vi "CalculateBMonly.vi"() -> ()   [LabVIEW 2016]
uses:
  <vilib>/Analysis/baseanly.llb/Mean (DBL).vi
  <vilib>/Utility/file.llb/Read Delimited Spreadsheet (string).vi
  <vilib>/Utility/file.llb/Write Delimited Spreadsheet (DBL).vi
  <vilib>/Analysis/NI_AALBase.lvlib
panel:
  in  "Save XY plot":bool
  out "XYplot":path
  in  "complete":bool
  in  "recalculate":bool
  in  "Save BM":bool
  out "good aoi":i32[](array[numeric])
  out "yBM":dbl[](array[numeric])
  out "xBM":dbl[](array[numeric])
  in  "Tab Control":enum32{"Files data", "Each file data"}(tab)
  out "N=":i32
  out "Filenames":string[](array[string])
  out "# of Frames":dbl[](array[numeric])
  out "# of AOI":dbl[](array[numeric])
  out "useful AOIs":dbl[](array[numeric])
  out "% of useful AOIs":dbl
  out "tt # of useful AOIs":i32
  out "tt # of AOIs":i32
  out "?":T1(graph)
  out "Xm=":dbl format="%0.2f"
  out "Ym=":dbl format="%0.2f"
  in  "Intervals":i32=10
  out "?":T1(graph)
  out "useful Aois (each file)":i32
  out "XY plot":T2
  in  "mode":enum32{"slide by slide", "delay"}(tab)=enum."delay"
  in  "next":bool
  in  "Run over":bool
  in  "second":dbl
  in  "run over":bool
  out "File":string
  in  "nm/pixel":dbl=72.5
  in  "±":dbl=50.0
  in  "BM":dbl=50.0
  out "BM lower limit":dbl
  out "BM upper limit":dbl
  in  "R should less than":dbl=0.2
  in  "lower limit":dbl=0.85
  in  "upper limit":dbl=1.15
  in  "BM range":bool=TRUE
  in  "Relation coefficient":bool
  in  "rotate?":bool
  in  "x/y":bool=TRUE
  out "all y position\n(pixel)":dbl[][](array[numeric])
  out "all x position\n(pixel)":dbl[][](array[numeric])
  out "# of frames":dbl
  out "# of AOIs":dbl
  out "Tandem Yi position":dbl[](array[numeric])
  out "Tandem Xi position":dbl[](array[numeric])
  out "path out":path
  in  "Path Folder":path
  out "XY Graph 2":cluster{dbl[], dbl[]}(graph)
  # "nm"
  # "nm"
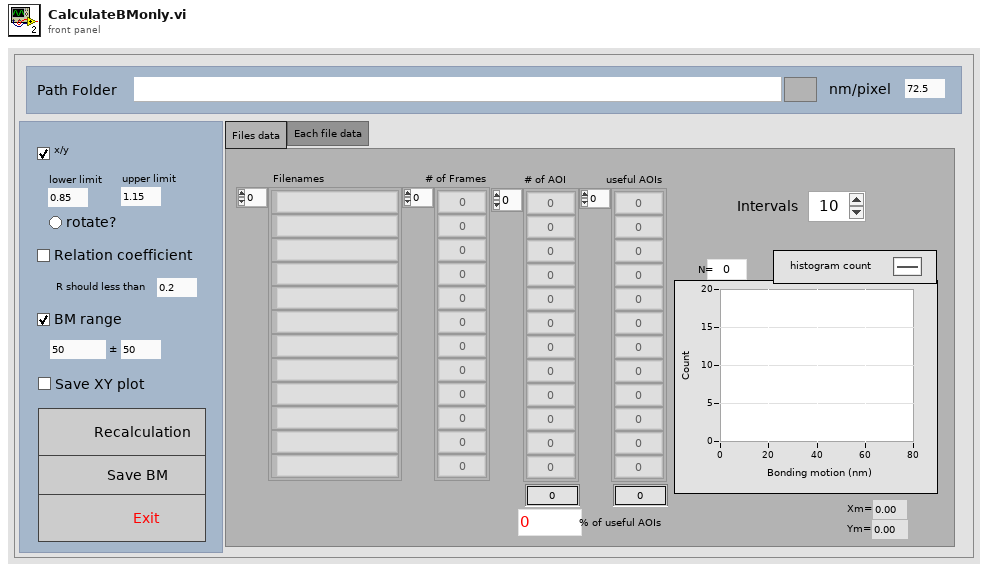
[diagram p1: front panel]
types:
  T1 = cluster{"X Values":dbl[], "Histogram: h(x)":i32[]}
  T2 = cluster{" X-Y plot":cluster{dbl[], dbl[]}, "Aoi":i32, "X BM":dbl, "Y BM":dbl}
  T3 = cluster{cluster{dbl[], dbl[]}, i32, "x standard deviation":dbl, "y standard deviation":dbl}
  T4 = typedef "imagedata.ctl" = cluster{"image type":i32, "image depth":i32, "image":u8[], "mask":u8[], "colors":u32[], "Rectangle":cluster{"left":i16, "top":i16, "right":i16, "bottom":i16}}
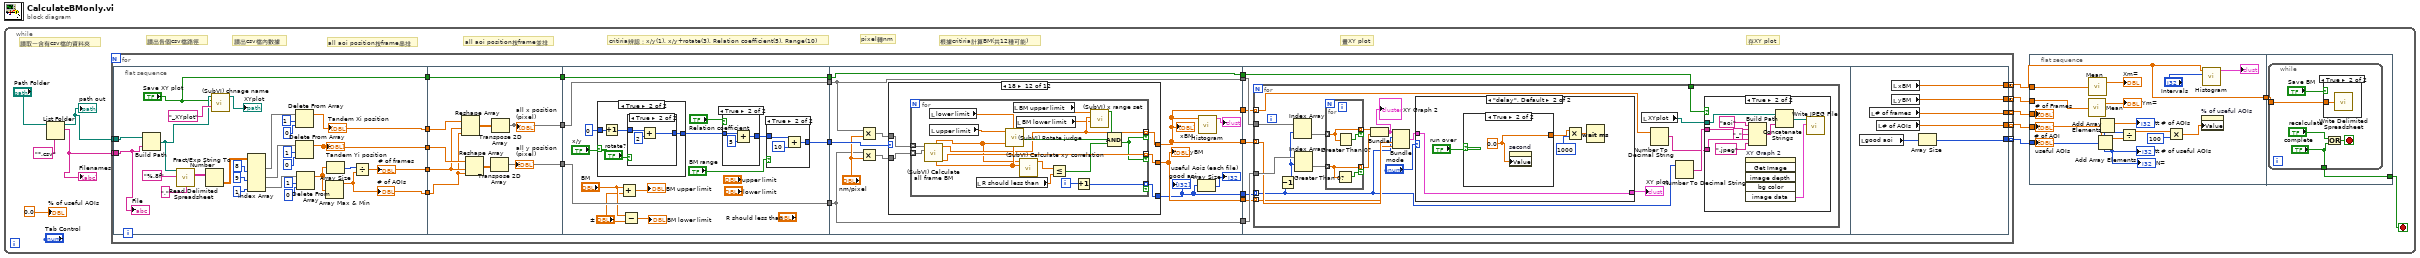
[diagram p0: block diagram]
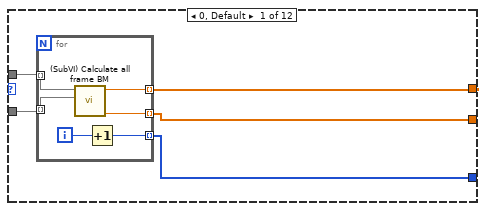
[diagram p7: hidden frame]
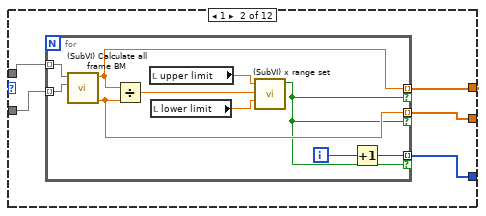
[diagram p8: hidden frame]
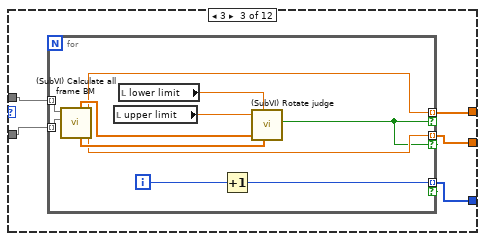
[diagram p9: hidden frame]
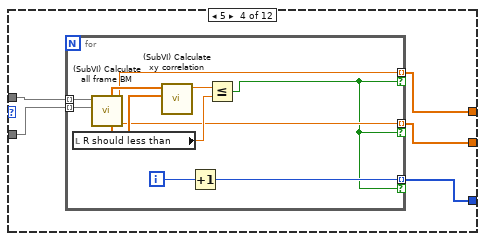
[diagram p10: hidden frame]
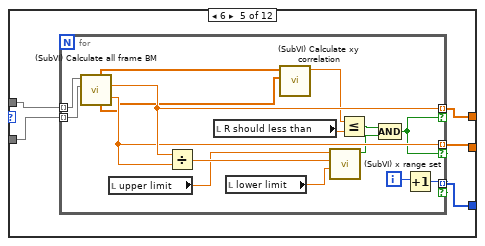
[diagram p11: hidden frame]
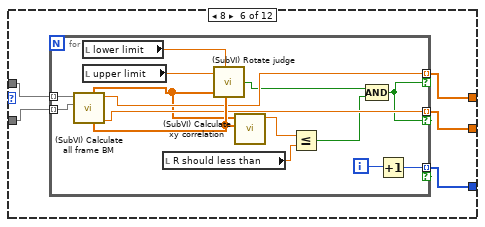
[diagram p12: hidden frame]
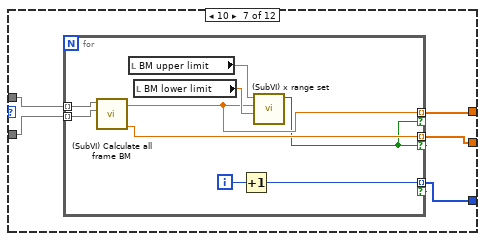
[diagram p13: hidden frame]
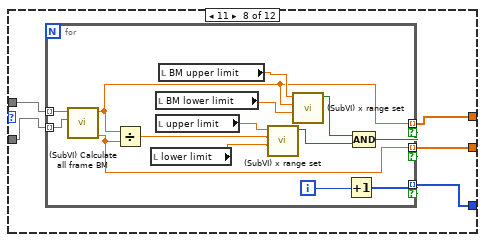
[diagram p14: hidden frame]
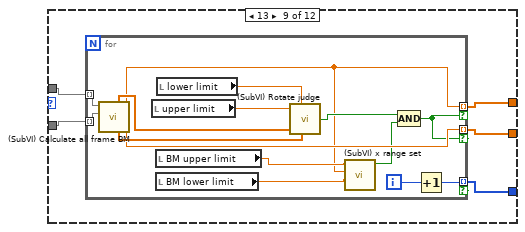
[diagram p15: hidden frame]
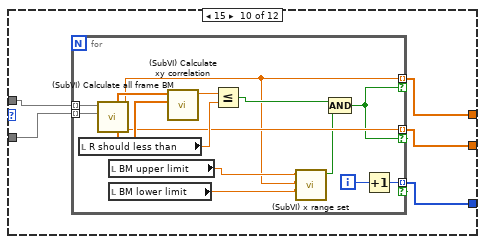
[diagram p16: hidden frame]
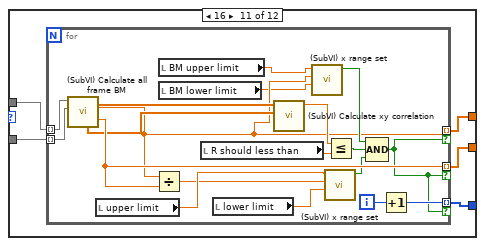
[diagram p17: hidden frame]
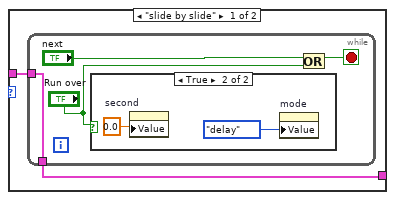
[diagram p19: hidden frame]
diagram:
  n1 = while {
    stop <- w2 stop-if-true
    # "存XY plot"
    # "畫XY plot"
    # "pixel轉nm"
    # "根據critiria計算BM(共12種可能)"
    # "critiria辨認：x/y(1), x/y+rotate(3), Relation coefficient(5), Range(10)"
    # "all aoi position按frame並排"
    # "all aoi position按frame串排"
    # "讀出csv檔內數據"
    # "讀出各個csv檔路徑"
    # "讀取一含有csv檔的資料夾"
    n2 = List Folder(path="Path Folder", pattern="*.csv") -> (path out=w9:path, filenames=w3:string[])  [unwired: 2 in, 2 out]
    "path out" <- w9
    "Filenames" <- w3
    n3 = for {
      tunnel: w9 -> [w51]
      tunnel: w3 -> [w50] mode=indexing
      tunnel: [w49] -> w4 mode=concatenating
      tunnel: [w48] -> w7 mode=concatenating
      tunnel: [w44] -> w5 mode=indexing
      tunnel: [w43] -> w8 mode=indexing
      tunnel: [w42] -> w6 mode=indexing
      n4 = flat-sequence {
        tunnel: [w88] -> w60
        tunnel: [w87] -> w59
        tunnel: [w86] -> w58
        tunnel: [w85] -> w57
        tunnel: w51 -> [w84]
        tunnel: w50 -> [w65]
        tunnel: ["Save XY plot"] -> w37
        tunnel: w60 -> [w97]
        tunnel: w59 -> [w96]
        tunnel: w58 -> [w95]
        tunnel: w57 -> [w94]
        tunnel: [w93] -> w56
        tunnel: [w92] -> w55
        tunnel: [w89] -> w38
        tunnel: w37 -> [w89]
        tunnel: w56 -> [w104]
        tunnel: w55 -> [w103]
        tunnel: [w105] -> w54
        tunnel: [w104] -> w53
        tunnel: [w103] -> w52
        tunnel: [w98] -> w39
        tunnel: w38 -> [w98]
        tunnel: w54 -> [w140]
        tunnel: w53 -> [w136]
        tunnel: w52 -> [w135]
        tunnel: [w130] -> w47
        tunnel: [w136] -> w46
        tunnel: [w135] -> w45
        tunnel: [w132] -> w41
        tunnel: [w134] -> w40
        tunnel: w39 -> [w133]
        tunnel: [w133] -> w36
        tunnel: [w132] -> w35
        tunnel: w40 -> [w362]
        tunnel: w41 -> [w363]
        tunnel: w45 -> [w365]
        tunnel: w46 -> [w366]
        tunnel: w47 -> [w364]
        tunnel: w36 -> [w361]
        tunnel: w35 -> [w360]
        tunnel: [w418] -> w48
        tunnel: [w419] -> w49
        tunnel: [w415] -> w44
        tunnel: [w417] -> w43
        tunnel: [w416] -> w42
        frame #0 {
          n5 = Build Path(base path=w84, name or relative path=w65) -> (appended path=w62:path)
          n6 = call-poly <vilib>:"Read Delimited Spreadsheet.vi"("file path (dialog if empty)"=w62, "format (%s)"="%.8f", "delimiter (\\t)"="," ("delimiter (\\t)")) -> ("all rows"=w81:string[][])  [unwired: 7 in, 5 out]
          n7 = Fract/Exp String To Number(string=w81) -> (number=w80:dbl[][])  [unwired: 3 in, 1 out]
          n8 = call "(SubVI) chnage name.vi"("replace \".csv\" to"="_XYplot" ("replace string (\"\")"), "Create path?"="Save XY plot", "Folder path"=w62) -> ("created path"=→"XYplot":path)  [unwired: 8 in]
          n9 = Index Array(array=w80, index (col) #1=8 ("disabled index (col)"), index (col) #2=9 ("index (col)"), index (col) #3=1 ("index (col)")) -> (element #1=w70:dbl[], element #2=w69:dbl[], element #3=w68:dbl[])  [unwired: 3 in]
          n10 = Delete From Array(array=w70, length=1, index=0) -> (array with subset deleted=w88:dbl[])  [unwired: 1 out]
          "Tandem Xi position" <- w88
          n11 = Delete From Array(array=w69, length=1, index=0) -> (array with subset deleted=w87:dbl[])  [unwired: 1 out]
          "Tandem Yi position" <- w87
          n12 = Delete From Array(array=w68, length=1, index=0) -> (array with subset deleted=w67:dbl[])  [unwired: 1 out]
          n13 = Array Max & Min(array=w67) -> (max value=w85:dbl)  [unwired: 3 out]
          "# of AOIs" <- w85
          n14 = Array Size(array=w67) -> (size(s)=w66:i32)
          n15 = Divide(x=w66, y=w85) -> (x/y=w86:dbl)
          "# of frames" <- w86
          "File" <- w65
        }
        frame #1 {
          n16 = Reshape Array(w97, w95, w94) -> (w91:dbl[][])
          n17 = Reshape Array(w96, w95, w94) -> (w90:dbl[][])
          n18 = Transpose 2D Array(2D array=w90) -> (transposed array=w92:dbl[][])
          "all y position\n(pixel)" <- w92
          n19 = Transpose 2D Array(2D array=w91) -> (transposed array=w93:dbl[][])
          "all x position\n(pixel)" <- w93
        }
        frame #2 {
          n20 = case shown="True" "x/y" {
            tunnel: 0 -> [w120 w124]
            tunnel: [w120 w121] -> w108
            frame False {
            }
            frame True {
              n21 = Increment(x=w124) -> (x+1=w122:i32)
              n22 = case shown="True" "rotate?" {
                tunnel: w122 -> [w125 w127]
                tunnel: [w125 w126] -> w121
                frame False {
                }
                frame True {
                  n23 = Add(x=w127, y=2) -> (x+y=w126:i32)
                }
              }
            }
          }
          n24 = Add(x="BM", y="±") -> (x+y=→"BM upper limit":dbl)
          n25 = Subtract(x="BM", y="±") -> (x-y=→"BM lower limit":dbl)
          n26 = case shown="True" "Relation coefficient" {
            tunnel: w108 -> [w116 w118]
            tunnel: [w116 w117] -> w111
            frame False {
            }
            frame True {
              n27 = Add(x=w118, y=5) -> (x+y=w117:i32)
            }
          }
          n28 = case shown="True" "BM range" {
            tunnel: w111 -> [w112 w114]
            tunnel: [w112 w113] -> w105
            frame False {
            }
            frame True {
              n29 = Add(x=w114, y=10) -> (x+y=w113:i32)
            }
          }
        }
        frame #3 {
          n30 = Multiply(x=w136, y="nm/pixel") -> (x*y=w138:dbl[][])
          n31 = Multiply(x=w135, y="nm/pixel") -> (x*y=w137:dbl[][])
          n32 = case shown="18" w140 {
            tunnel: w138 -> [w145 w156 w171 w187 w203 w224 w244 w258 w277 w297 w317 w341]
            tunnel: w137 -> [w144 w155 w170 w186 w202 w223 w243 w257 w276 w296 w316 w340]
            tunnel: [w143 w154 w169 w185 w201 w222 w242 w256 w275 w295 w315 w339] -> w132
            tunnel: [w142 w153 w168 w184 w200 w221 w241 w255 w274 w294 w314 w338] -> w134
            tunnel: [w141 w152 w167 w183 w199 w220 w240 w254 w273 w293 w313 w337] -> w130
            frame 0, Default {
              n33 = for {
                tunnel: w145 -> [w151] mode=indexing
                tunnel: w144 -> [w150] mode=indexing
                tunnel: [w149] -> w143 mode=indexing
                tunnel: [w148] -> w142 mode=indexing
                tunnel: [w146] -> w141 mode=indexing
                i -> [w147]
                n34 = call "(SubVI) Calculate all frame BM.vi"("y position (pixel)"=w150, "x position (pixel)"=w151) -> ("y standard deviation"=w148:dbl, "x standard deviation"=w149:dbl)  [unwired: 6 in, 2 out]
                n35 = Increment(x=w147) -> (x+1=w146:i32)
              }
            }
            frame 1 {
              n36 = for {
                tunnel: [w166] -> w154 mode=indexing if=w158
                tunnel: [w165] -> w153 mode=indexing if=w158
                tunnel: w156 -> [w164] mode=indexing
                tunnel: w155 -> [w163] mode=indexing
                tunnel: [w157] -> w152 mode=indexing if=w158
                i -> [w159]
                n37 = call "(SubVI) Calculate all frame BM.vi"("y position (pixel)"=w163, "x position (pixel)"=w164) -> ("y standard deviation"=w165:dbl, "x standard deviation"=w166:dbl)  [unwired: 6 in, 2 out]
                n38 = Divide(x=w166, y=w165) -> (x/y=w161:dbl)
                n39 = local read "upper limit"() -> (w162:dbl)
                n40 = local read "lower limit"() -> (w160:dbl)
                n41 = call "(SubVI) x range set.vi"("lower limit"=w160, "x"=w161, "upper limit"=w162) -> ("Boolean"=w158:bool)  [unwired: 8 in]
                n42 = Increment(x=w159) -> (x+1=w157:i32)
              }
            }
            frame 3 {
              n43 = for {
                tunnel: w171 -> [w182] mode=indexing
                tunnel: w170 -> [w181] mode=indexing
                tunnel: [w176] -> w169 mode=indexing if=w172
                tunnel: [w175] -> w168 mode=indexing if=w172
                tunnel: [w173] -> w167 mode=indexing if=w172
                i -> [w174]
                n44 = call "(SubVI) Calculate all frame BM.vi"("y position (pixel)"=w181, "x position (pixel)"=w182) -> ("y standard deviation"=w175:dbl, "x standard deviation"=w176:dbl, "y position (delete y fit error)"=w179:dbl[], "x position (delete x fit error)"=w180:dbl[])  [unwired: 6 in]
                n45 = local read "upper limit"() -> (w178:dbl)
                n46 = local read "lower limit"() -> (w177:dbl)
                n47 = Increment(x=w174) -> (x+1=w173:i32)
                n48 = call "(SubVI) Rotate judge.vi"("x/y upper limit"=w178, "x/y lower limit"=w177, "x position (delete y fit error)"=w180, "y position (delete y fit error)"=w179) -> ("x = y?"=w172:bool)  [unwired: 1 in]
              }
            }
            frame 5 {
              n49 = for {
                tunnel: w187 -> [w198] mode=indexing
                tunnel: w186 -> [w197] mode=indexing
                tunnel: [w192] -> w185 mode=indexing if=w188
                tunnel: [w191] -> w184 mode=indexing if=w188
                tunnel: [w189] -> w183 mode=indexing if=w188
                i -> [w190]
                n50 = local read "R should less than"() -> (w193:dbl)
                n51 = call "(SubVI) Calculate all frame BM.vi"("y position (pixel)"=w197, "x position (pixel)"=w198) -> ("y standard deviation"=w191:dbl, "x standard deviation"=w192:dbl, "y position (delete y fit error)"=w195:dbl[], "x position (delete x fit error)"=w196:dbl[])  [unwired: 6 in]
                n52 = call "(SubVI) Calculate xy correlation.vi"("y position (delete y fit error)"=w195, "x position (delete x fit error)"=w196) -> ("Numeric"=w194:dbl)  [unwired: 9 in]
                n53 = Increment(x=w190) -> (x+1=w189:i32)
                n54 = Less Or Equal?(x=w194, y=w193) -> (x <= y?=w188:bool)
              }
            }
            frame 6 {
              n55 = for {
                tunnel: w203 -> [w219] mode=indexing
                tunnel: w202 -> [w218] mode=indexing
                tunnel: [w217] -> w201 mode=indexing if=w204
                tunnel: [w216] -> w200 mode=indexing if=w204
                tunnel: [w205] -> w199 mode=indexing if=w204
                i -> [w206]
                n56 = call "(SubVI) Calculate all frame BM.vi"("y position (pixel)"=w218, "x position (pixel)"=w219) -> ("y standard deviation"=w216:dbl, "x standard deviation"=w217:dbl, "y position (delete y fit error)"=w212:dbl[], "x position (delete x fit error)"=w213:dbl[])  [unwired: 6 in]
                n57 = local read "upper limit"() -> (w208:dbl)
                n58 = Divide(x=w217, y=w216) -> (x/y=w209:dbl)
                n59 = local read "R should less than"() -> (w214:dbl)
                n60 = local read "lower limit"() -> (w207:dbl)
                n61 = call "(SubVI) Calculate xy correlation.vi"("y position (delete y fit error)"=w212, "x position (delete x fit error)"=w213) -> ("Numeric"=w215:dbl)  [unwired: 9 in]
                n62 = call "(SubVI) x range set.vi"("lower limit"=w207, "x"=w209, "upper limit"=w208) -> ("Boolean"=w211:bool)  [unwired: 8 in]
                n63 = Less Or Equal?(x=w215, y=w214) -> (x <= y?=w210:bool)
                n64 = Compound Arithmetic op=AND(w210, w211) -> (w204:bool)
                n65 = Increment(x=w206) -> (x+1=w205:i32)
              }
            }
            frame 8 {
              n66 = for {
                tunnel: w224 -> [w239] mode=indexing
                tunnel: w223 -> [w238] mode=indexing
                tunnel: [w232] -> w222 mode=indexing if=w226
                tunnel: [w231] -> w221 mode=indexing if=w226
                tunnel: [w227] -> w220 mode=indexing if=w226
                i -> [w228]
                n67 = call "(SubVI) Calculate all frame BM.vi"("y position (pixel)"=w238, "x position (pixel)"=w239) -> ("y standard deviation"=w231:dbl, "x standard deviation"=w232:dbl, "y position (delete y fit error)"=w237:dbl[], "x position (delete x fit error)"=w225:dbl[])  [unwired: 6 in]
                n68 = local read "lower limit"() -> (w235:dbl)
                n69 = local read "upper limit"() -> (w236:dbl)
                n70 = local read "R should less than"() -> (w233:dbl)
                n71 = call "(SubVI) Rotate judge.vi"("x/y upper limit"=w236, "x/y lower limit"=w235, "x position (delete y fit error)"=w225, "y position (delete y fit error)"=w237) -> ("x = y?"=w230:bool)  [unwired: 1 in]
                n72 = call "(SubVI) Calculate xy correlation.vi"("y position (delete y fit error)"=w237, "x position (delete x fit error)"=w225) -> ("Numeric"=w234:dbl)  [unwired: 9 in]
                n73 = Less Or Equal?(x=w234, y=w233) -> (x <= y?=w229:bool)
                n74 = Compound Arithmetic op=AND(w230, w229) -> (w226:bool)
                n75 = Increment(x=w228) -> (x+1=w227:i32)
              }
            }
            frame 10 {
              n76 = for {
                tunnel: w244 -> [w253] mode=indexing
                tunnel: w243 -> [w252] mode=indexing
                tunnel: [w248] -> w242 mode=indexing if=w245
                tunnel: [w251] -> w241 mode=indexing if=w245
                tunnel: [w246] -> w240 mode=indexing if=w245
                i -> [w247]
                n77 = call "(SubVI) Calculate all frame BM.vi"("y position (pixel)"=w252, "x position (pixel)"=w253) -> ("y standard deviation"=w251:dbl, "x standard deviation"=w248:dbl)  [unwired: 6 in, 2 out]
                n78 = local read "BM upper limit"() -> (w250:dbl)
                n79 = local read "BM lower limit"() -> (w249:dbl)
                n80 = Increment(x=w247) -> (x+1=w246:i32)
                n81 = call "(SubVI) x range set.vi"("lower limit"=w249, "x"=w248, "upper limit"=w250) -> ("Boolean"=w245:bool)  [unwired: 8 in]
              }
            }
            frame 11 {
              n82 = for {
                tunnel: w258 -> [w272] mode=indexing
                tunnel: w257 -> [w271] mode=indexing
                tunnel: [w267] -> w256 mode=indexing if=w259
                tunnel: [w270] -> w255 mode=indexing if=w259
                tunnel: [w260] -> w254 mode=indexing if=w259
                i -> [w261]
                n83 = call "(SubVI) Calculate all frame BM.vi"("y position (pixel)"=w271, "x position (pixel)"=w272) -> ("y standard deviation"=w270:dbl, "x standard deviation"=w267:dbl)  [unwired: 6 in, 2 out]
                n84 = Divide(x=w267, y=w270) -> (x/y=w263:dbl)
                n85 = local read "lower limit"() -> (w262:dbl)
                n86 = local read "BM lower limit"() -> (w266:dbl)
                n87 = local read "upper limit"() -> (w265:dbl)
                n88 = local read "BM upper limit"() -> (w268:dbl)
                n89 = call "(SubVI) x range set.vi"("lower limit"=w262, "x"=w263, "upper limit"=w265) -> ("Boolean"=w264:bool)  [unwired: 8 in]
                n90 = call "(SubVI) x range set.vi"("lower limit"=w266, "x"=w267, "upper limit"=w268) -> ("Boolean"=w269:bool)  [unwired: 8 in]
                n91 = Increment(x=w261) -> (x+1=w260:i32)
                n92 = Compound Arithmetic op=AND(w269, w264) -> (w259:bool)
              }
            }
            frame 13 {
              n93 = for {
                tunnel: w277 -> [w292] mode=indexing
                tunnel: w276 -> [w291] mode=indexing
                tunnel: [w282] -> w275 mode=indexing if=w278
                tunnel: [w286] -> w274 mode=indexing if=w278
                tunnel: [w279] -> w273 mode=indexing if=w278
                i -> [w280]
                n94 = call "(SubVI) Calculate all frame BM.vi"("y position (pixel)"=w291, "x position (pixel)"=w292) -> ("y standard deviation"=w286:dbl, "x standard deviation"=w282:dbl, "y position (delete y fit error)"=w289:dbl[], "x position (delete x fit error)"=w290:dbl[])  [unwired: 6 in]
                n95 = local read "upper limit"() -> (w288:dbl)
                n96 = local read "BM upper limit"() -> (w283:dbl)
                n97 = local read "BM lower limit"() -> (w281:dbl)
                n98 = local read "lower limit"() -> (w287:dbl)
                n99 = call "(SubVI) Rotate judge.vi"("x/y upper limit"=w288, "x/y lower limit"=w287, "x position (delete y fit error)"=w290, "y position (delete y fit error)"=w289) -> ("x = y?"=w285:bool)  [unwired: 1 in]
                n100 = call "(SubVI) x range set.vi"("lower limit"=w281, "x"=w282, "upper limit"=w283) -> ("Boolean"=w284:bool)  [unwired: 8 in]
                n101 = Compound Arithmetic op=AND(w285, w284) -> (w278:bool)
                n102 = Increment(x=w280) -> (x+1=w279:i32)
              }
            }
            frame 15 {
              n103 = for {
                tunnel: w297 -> [w312] mode=indexing
                tunnel: w296 -> [w311] mode=indexing
                tunnel: [w302] -> w295 mode=indexing if=w298
                tunnel: [w306] -> w294 mode=indexing if=w298
                tunnel: [w299] -> w293 mode=indexing if=w298
                i -> [w300]
                n104 = local read "R should less than"() -> (w307:dbl)
                n105 = call "(SubVI) Calculate all frame BM.vi"("y position (pixel)"=w311, "x position (pixel)"=w312) -> ("y standard deviation"=w306:dbl, "x standard deviation"=w302:dbl, "y position (delete y fit error)"=w309:dbl[], "x position (delete x fit error)"=w310:dbl[])  [unwired: 6 in]
                n106 = local read "BM upper limit"() -> (w303:dbl)
                n107 = local read "BM lower limit"() -> (w301:dbl)
                n108 = call "(SubVI) Calculate xy correlation.vi"("y position (delete y fit error)"=w309, "x position (delete x fit error)"=w310) -> ("Numeric"=w308:dbl)  [unwired: 9 in]
                n109 = Less Or Equal?(x=w308, y=w307) -> (x <= y?=w305:bool)
                n110 = call "(SubVI) x range set.vi"("lower limit"=w301, "x"=w302, "upper limit"=w303) -> ("Boolean"=w304:bool)  [unwired: 8 in]
                n111 = Compound Arithmetic op=AND(w305, w304) -> (w298:bool)
                n112 = Increment(x=w300) -> (x+1=w299:i32)
              }
            }
            frame 16 {
              n113 = for {
                tunnel: w317 -> [w336] mode=indexing
                tunnel: w316 -> [w335] mode=indexing
                tunnel: [w326] -> w315 mode=indexing if=w318
                tunnel: [w334] -> w314 mode=indexing if=w318
                tunnel: [w319] -> w313 mode=indexing if=w318
                i -> [w320]
                n114 = call "(SubVI) Calculate all frame BM.vi"("y position (pixel)"=w335, "x position (pixel)"=w336) -> ("y standard deviation"=w334:dbl, "x standard deviation"=w326:dbl, "y position (delete y fit error)"=w330:dbl[], "x position (delete x fit error)"=w331:dbl[])  [unwired: 6 in]
                n115 = local read "upper limit"() -> (w323:dbl)
                n116 = Divide(x=w326, y=w334) -> (x/y=w322:dbl)
                n117 = local read "BM upper limit"() -> (w327:dbl)
                n118 = local read "BM lower limit"() -> (w325:dbl)
                n119 = local read "R should less than"() -> (w332:dbl)
                n120 = local read "lower limit"() -> (w321:dbl)
                n121 = call "(SubVI) Calculate xy correlation.vi"("y position (delete y fit error)"=w330, "x position (delete x fit error)"=w331) -> ("Numeric"=w333:dbl)  [unwired: 9 in]
                n122 = call "(SubVI) x range set.vi"("lower limit"=w325, "x"=w326, "upper limit"=w327) -> ("Boolean"=w328:bool)  [unwired: 8 in]
                n123 = call "(SubVI) x range set.vi"("lower limit"=w321, "x"=w322, "upper limit"=w323) -> ("Boolean"=w324:bool)  [unwired: 8 in]
                n124 = Less Or Equal?(x=w333, y=w332) -> (x <= y?=w329:bool)
                n125 = Compound Arithmetic op=AND(w328, w329, w324) -> (w318:bool)
                n126 = Increment(x=w320) -> (x+1=w319:i32)
              }
            }
            frame 18 {
              n127 = for {
                tunnel: w341 -> [w359] mode=indexing
                tunnel: w340 -> [w358] mode=indexing
                tunnel: [w347] -> w339 mode=indexing if=w343
                tunnel: [w352] -> w338 mode=indexing if=w343
                tunnel: [w344] -> w337 mode=indexing if=w343
                i -> [w345]
                n128 = call "(SubVI) Calculate all frame BM.vi"("y position (pixel)"=w358, "x position (pixel)"=w359) -> ("y standard deviation"=w352:dbl, "x standard deviation"=w347:dbl, "y position (delete y fit error)"=w357:dbl[], "x position (delete x fit error)"=w342:dbl[])  [unwired: 6 in]
                n129 = local read "lower limit"() -> (w355:dbl)
                n130 = local read "upper limit"() -> (w356:dbl)
                n131 = local read "R should less than"() -> (w353:dbl)
                n132 = call "(SubVI) Rotate judge.vi"("x/y upper limit"=w356, "x/y lower limit"=w355, "x position (delete y fit error)"=w342, "y position (delete y fit error)"=w357) -> ("x = y?"=w351:bool)  [unwired: 1 in]
                n133 = local read "BM upper limit"() -> (w348:dbl)
                n134 = local read "BM lower limit"() -> (w346:dbl)
                n135 = call "(SubVI) Calculate xy correlation.vi"("y position (delete y fit error)"=w357, "x position (delete x fit error)"=w342) -> ("Numeric"=w354:dbl)  [unwired: 9 in]
                n136 = Less Or Equal?(x=w354, y=w353) -> (x <= y?=w350:bool)
                n137 = Increment(x=w345) -> (x+1=w344:i32)
                n138 = call "(SubVI) x range set.vi"("lower limit"=w346, "x"=w347, "upper limit"=w348) -> ("Boolean"=w349:bool)  [unwired: 8 in]
                n139 = Compound Arithmetic op=AND(w349, w351, w350) -> (w343:bool)
              }
            }
          }
          "xBM" <- w132
          "yBM" <- w134
          "good aoi" <- w130
          n140 = Array Size(array=w130) -> (size(s)=→"useful Aois (each file)":i32)
          n141 = call <vilib>:"Histogram.vi"("X"=w132) -> ("Histogram Graph"=→"?":T1)  [unwired: 7 in, 3 out]
        }
        frame #4 {
          n142 = for {
            tunnel: w366 -> [w385]
            tunnel: w365 -> [w384]
            tunnel: w364 -> [w369] mode=indexing
            tunnel: w363 -> [w383] mode=indexing
            tunnel: w362 -> [w382] mode=indexing
            tunnel: w361 -> [w370]
            tunnel: w360 -> [w368] mode=indexing
            n143 = Decrement(x=w369) -> (x-1=w376:i32)
            n144 = Index Array(array=w385, index (row)=w376) -> (element=w379:dbl[])  [unwired: 1 in]
            n145 = Index Array(array=w384, index (row)=w376) -> (element=w378:dbl[])  [unwired: 1 in]
            n146 = for {
              tunnel: w379 -> [w413] mode=indexing
              tunnel: w378 -> [w412] mode=indexing
              tunnel: [w413] -> w381 mode=indexing if=w411
              tunnel: [w412] -> w380 mode=indexing if=w410
              n147 = Greater Than 0?(x=w412) -> (x > 0?=w410:bool)
              n148 = Greater Than 0?(x=w413) -> (x > 0?=w411:bool)
            }
            n149 = Bundle(w381, w380) -> (w374:cluster{dbl[], dbl[]})  [unwired: 1 in]
            "XY Graph 2" <- w374
            n150 = Bundle(w374, w369, "x standard deviation"=w383, "y standard deviation"=w382) -> (w377:T3)  [unwired: 1 in]
            n151 = case shown="\"delay\", Default" "mode" {
              tunnel: w377 -> [w396 w404]
              tunnel: [w395 w404] -> w367
              frame "slide by slide" {
                n152 = while {
                  tunnel: w396 -> [w399]
                  tunnel: [w399] -> w395
                  stop <- w398 stop-if-true
                  n153 = case shown="True" "Run over" {
                    frame False {
                    }
                    frame True {
                      n154 = property on="second" class="DigNum (strict)"("Value"=0.0 ("seconds to wait")) -> ()  [unwired: 2 in, 2 out]
                      n155 = property on="mode" class="TabCtl (strict)"("Value"=enum32{"slide by slide", "delay"}."delay" ("mode")) -> ()  [unwired: 2 in, 2 out]
                    }
                  }
                  n156 = Or(x="next", y="Run over") -> (x .or. y?=w398:bool)
                }
              }
              frame "delay", Default {
                n157 = case shown="True" "run over" {
                  tunnel: ["second" w409] -> w405
                  frame False {
                  }
                  frame True {
                    w409 = 0.0
                    n158 = property on="second" class="DigNum (strict)"("Value"=w409) -> ()  [unwired: 2 in, 2 out]
                  }
                }
                n159 = Multiply(x=w405, y=u32 1000) -> (x*y=w406:dbl)
                n160 = Wait (ms)(milliseconds to wait=w406) -> ()  [unwired: 1 out]
              }
            }
            "XY plot" <- w367
            n161 = local read "XYplot"() -> (w371:path)
            n162 = Number To Decimal String(number=w368) -> (decimal integer string=w372:string)  [unwired: 1 in]
            n163 = Number To Decimal String(number=w369) -> (decimal integer string=w373:string)  [unwired: 1 in]
            n164 = case shown="True" w370 {
              tunnel: w373 -> [_ w394]
              tunnel: w371 -> [_ w392]
              tunnel: w372 -> [_ w387]
              frame False {
              }
              frame True {
                n165 = invoke on="XY Graph 2" class="XYGraph (strict)" method="Get Image"() -> ("image data"=w386:T4)  [unwired: 6 in, 5 out]
                n166 = Concatenate Strings("aoi" ("string"), w394, "_" ("string"), w387, ".jpeg" ("string")) -> (w393:string)
                n167 = Build Path(base path=w392, name or relative path=w393) -> (appended path=w391:path)
                n168 = call <vilib>:"Write JPEG File.vi"("image data"=w386, "path to JPEG file"=w391) -> ()  [unwired: 8 in, 2 out]
              }
            }
          }
        }
        frame #5 {
          n169 = local read "good aoi"() -> (w414:i32[])
          n170 = local read "# of frames"() -> (w417:dbl)
          n171 = local read "# of AOIs"() -> (w416:dbl)
          n172 = local read "xBM"() -> (w419:dbl[])
          n173 = local read "yBM"() -> (w418:dbl[])
          n174 = Array Size(array=w414) -> (size(s)=w415:i32)
        }
      }
    }
    n175 = flat-sequence {
      tunnel: w8 -> [w26]
      tunnel: w7 -> [w25]
      tunnel: w6 -> [w22]
      tunnel: w5 -> [w21]
      tunnel: w4 -> [w15]
      tunnel: [w15] -> w12
      tunnel: w12 -> [w28]
      tunnel: [w27] -> w2
      frame #0 {
        n176 = call-poly <vilib>:"Mean.vi"("X"=w25) -> ("mean"=→"Ym=":dbl)  [unwired: 1 out]
        n177 = call-poly <vilib>:"Mean.vi"("X"=w15) -> ("mean"=→"Xm=":dbl)  [unwired: 1 out]
        n178 = Add Array Elements(numeric array=w21) -> (sum=w16:i32)
        "tt # of useful AOIs" <- w16
        "N=" <- w16
        n179 = Add Array Elements(numeric array=w22) -> (sum=w18:dbl)
        "tt # of AOIs" <- w18
        n180 = Divide(x=w16, y=w18) -> (x/y=w20:dbl)
        n181 = Multiply(x=w20, y=100) -> (x*y=w13:dbl)
        n182 = property on="% of useful AOIs" class="DigNum (strict)"("Value"=w13) -> ()  [unwired: 2 in, 2 out]
        n183 = call <vilib>:"Histogram.vi"("intervals"="Intervals", "X"=w15) -> ("Histogram Graph"=→"?":T1)  [unwired: 6 in, 3 out]
        "# of Frames" <- w26
        "useful AOIs" <- w21
        "# of AOI" <- w22
      }
      frame #1 {
        n184 = while {
          tunnel: w28 -> [w33]
          tunnel: ["complete"] -> w27
          stop <- w30 stop-if-true
          n185 = case shown="True" "Save BM" {
            tunnel: w33 -> [_ w34]
            frame False {
            }
            frame True {
              n186 = call-poly <vilib>:"Write Delimited Spreadsheet.vi"("1D data"=w34) -> ()  [unwired: 13 in, 2 out]
            }
          }
          n187 = Or(x="recalculate", y="complete") -> (x .or. y?=w30:bool)
        }
      }
    }
    "% of useful AOIs" <- 0.0
  }
